vi "API_Set_Finite_Time.vi"(1 "Finite Time":dbl, 2 "Argument List In":string[](array[string])) -> (0 "Argument List Out":string[](array[string]))   [LabVIEW 2011]
doc: "This VI takes the time value given by the user on the Growth Sequence Editor front panel, and appends it to the argument list. This value can also be set inside an API."
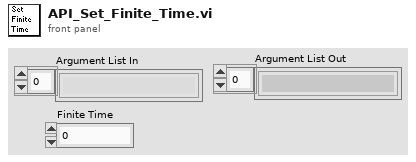
[diagram p1: front panel]
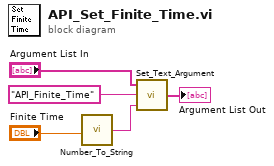
[diagram p0: block diagram]
diagram:
  n1 = call "Number_To_String.vi"("Number"="Finite Time") -> ("String"=w2:string)
  n2 = call "Set_Text_Argument.vi"("Text"=w2, "Argument"="API_Finite_Time", "Argument List In"="Argument List In") -> ("Argument List Out"=→"Argument List Out":string[])
